vi "Fermi Level Scan.vi"() -> ()   [LabVIEW 2018]
uses:
  <vilib>/Utility/file.llb/Write Delimited Spreadsheet (string).vi
  <vilib>/Utility/file.llb/Write Delimited Spreadsheet (DBL).vi
panel:
  out "?":bool
  in  "?":bool
  in  "Log Data?":bool
  out "Supply Voltage":dbl
  out "File Location":path
  out "Electron Energy (ev)":dbl
  out "error out":errorcluster
  out "Sample Current (A)":dbl
  in  "Voltage Increment (V)":dbl(knob) scale=0.0..1.0
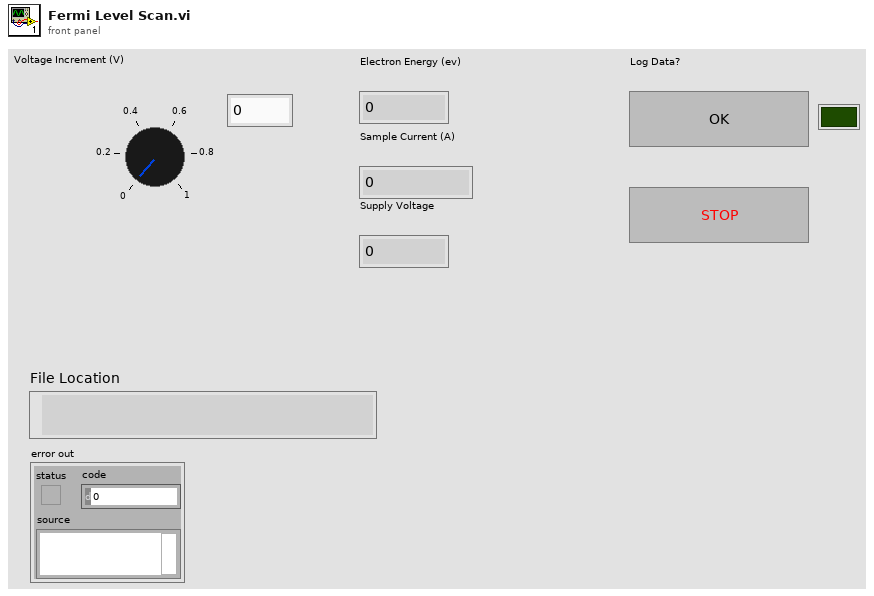
[diagram p1: front panel]
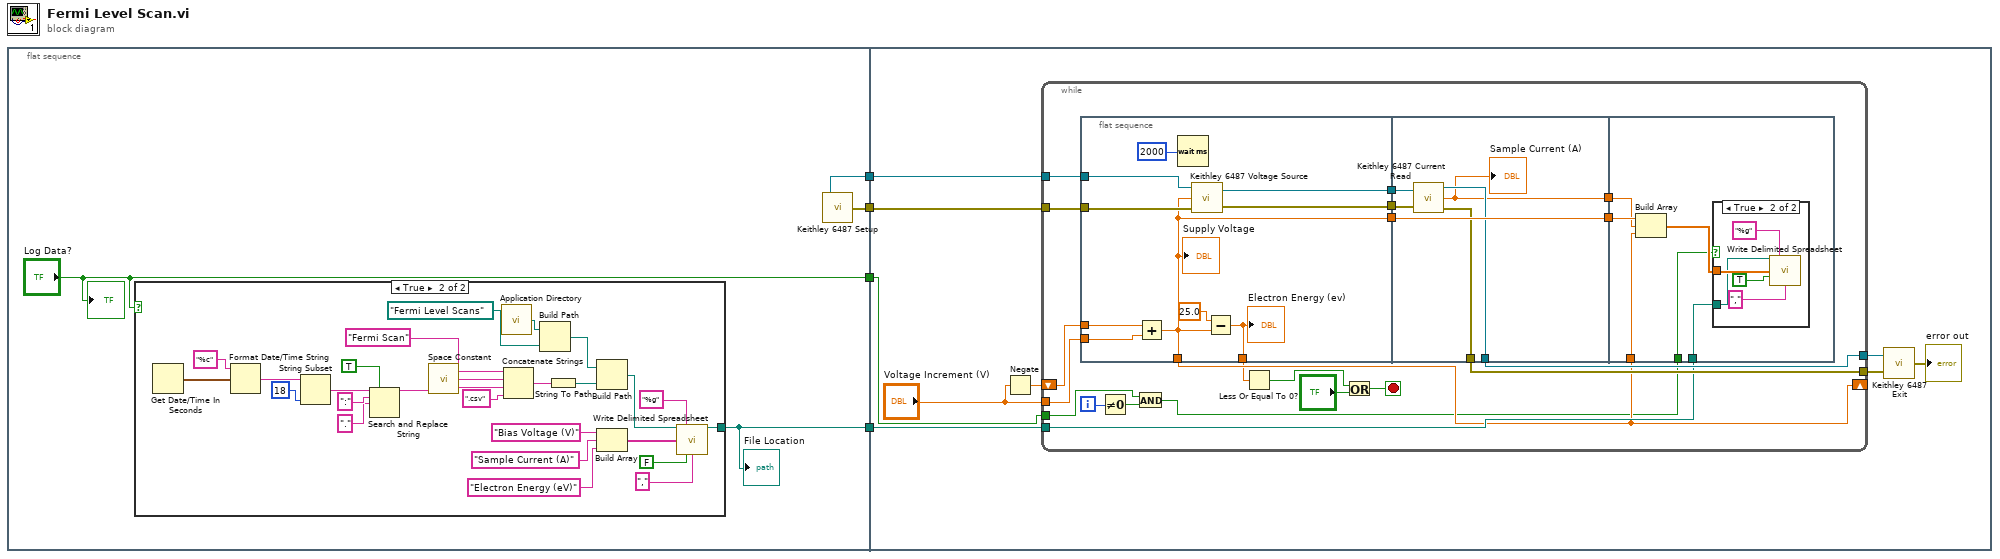
[diagram p0: block diagram]
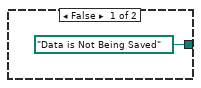
[diagram p2: hidden frame]
diagram:
  n1 = flat-sequence {
    tunnel: [w8] -> w4
    tunnel: [w6] -> w3
    tunnel: [w5] -> w2
    tunnel: ["Log Data?"] -> w1
    tunnel: w4 -> [w40]
    tunnel: w3 -> [w44]
    tunnel: w2 -> [w43]
    tunnel: w1 -> [w39]
    frame #0 {
      n2 = case shown="True" "Log Data?" {
        tunnel: [path "Data is Not Being Saved" ("new file path (Not A Path if cancelled)") w10] -> w8
        frame False {
        }
        frame True {
          n3 = Get Date/Time In Seconds() -> (seconds since 1Jan1904=w33:timestamp)
          n4 = Format Date/Time String(time format string (%c)="%c", seconds (now)=w33) -> (date/time string=w28:string)  [unwired: 1 in]
          n5 = String Subset(string=w28, length (rest)=18 ("length (rest)")) -> (substring=w29:string)  [unwired: 1 in]
          n6 = Search and Replace String(replace all?=TRUE, input string=w29, search string=":", replace string="." ("replace string (\"\")")) -> (result string=w24:string)  [unwired: 4 in, 3 out]
          n7 = call <vilib>:"Space Constant.vi"() -> ("String"=w25:string)
          n8 = call <vilib>:"Application Directory.vi"() -> ("Application Directory"=w17:path)
          n9 = Concatenate Strings("Fermi Scan", w25, w24, ".csv" ("string")) -> (w23:string)
          n10 = Build Path(base path=w17, name or relative path=path "Fermi Level Scans") -> (appended path=w34:path)
          n11 = String To Path(string=w23) -> (path=w22:path)
          n12 = Build Path(base path=w34, name or relative path=w22) -> (appended path=w21:path)
          n13 = Build Array("Bias Voltage (V)", "Sample Current (A)", "Electron Energy (eV)") -> (w12:string[])
          n14 = call-poly <vilib>:"Write Delimited Spreadsheet.vi"("file path (dialog if empty)"=w21, "format (%s)"="%g" ("format (%.3f)"), "1D data"=w12, "transpose? (no:F)"=FALSE, "delimiter (\\t)"="," ("delimiter (\\t)")) -> ("new file path (Not A Path if cancelled)"=w10:path)  [unwired: 9 in, 1 out]
        }
      }
      "File Location" <- w8
      n15 = call "Keithley 6487 Setup.vi"() -> ("error out"=w5:errorcluster, "VISA resource name out"=w6:refnum<visa-resource-name>)
      "?" <- "Log Data?"
    }
    frame #1 {
      n16 = Negate(x="Voltage Increment (V)") -> (-x=w41:dbl)
      n17 = while {
        tunnel: w44 -> [w65]
        tunnel: w43 -> [w64]
        shift-right: [w51] -> _
        shift-left: w41 -> [w61]
        tunnel: "Voltage Increment (V)" -> [w60]
        tunnel: [w58] -> w38
        tunnel: [w57] -> w37
        tunnel: w40 -> [w55]
        tunnel: w39 -> [w46]
        i -> [w48]
        stop <- w53 stop-if-true
        n18 = flat-sequence {
          tunnel: w65 -> [w68]
          tunnel: w64 -> [w69]
          tunnel: [w71] -> w63
          tunnel: [w70] -> w62
          tunnel: [w67] -> w51
          tunnel: w61 -> [w75]
          tunnel: w60 -> [w74]
          tunnel: [w67] -> w59
          tunnel: [w72] -> w50
          tunnel: w63 -> [w80]
          tunnel: w62 -> [w79]
          tunnel: w59 -> [w81]
          tunnel: [w78] -> w58
          tunnel: [w77] -> w57
          tunnel: [w81] -> w56
          tunnel: [w76] -> w52
          tunnel: w56 -> [w87]
          tunnel: w55 -> [w85]
          tunnel: w52 -> [w84]
          tunnel: w51 -> [w83]
          tunnel: w45 -> [w82]
          frame #0 {
            n19 = Add(x=w75, y=w74) -> (x+y=w67:dbl)
            "Supply Voltage" <- w67
            n20 = Wait (ms)(milliseconds to wait=u32 2000) -> ()  [unwired: 1 out]
            n21 = call "Keithley 6487 Voltage Source.vi"("error in (no error)"=w69, "Voltage"=w67, "VISA resource name"=w68) -> ("error out"=w70:errorcluster, "VISA resource name out"=w71:refnum<visa-resource-name>)
            n22 = Subtract(x=25.0, y=w67) -> (x-y=w72:dbl)
            "Electron Energy (ev)" <- w72
          }
          frame #1 {
            n23 = call "Keithley 6487 Current Read.vi"("VISA resource name"=w80, "error in (no error)"=w79) -> ("VISA out"=w78:refnum<visa-resource-name>, "Current (A)"=w76:dbl, "error out"=w77:errorcluster)
            "Sample Current (A)" <- w76
          }
          frame #2 {
            n24 = Build Array(w87, w84, w83) -> (w86:dbl[])
            n25 = case shown="True" w82 {
              tunnel: w86 -> [_ w92]
              tunnel: w85 -> [_ w91]
              frame False {
              }
              frame True {
                n26 = call-poly <vilib>:"Write Delimited Spreadsheet.vi"("file path (dialog if empty)"=w91, "format (%.3f)"="%g", "1D data"=w92, "append to file? (new file:F)"=TRUE, "delimiter (\\t)"="," ("delimiter (\\t)")) -> ()  [unwired: 9 in, 2 out]
              }
            }
          }
        }
        n27 = Not Equal To 0?(x=w48) -> (x != 0?=w47:bool)
        n28 = And(x=w46, y=w47) -> (x .and. y?=w45:bool)
        n29 = Less Or Equal To 0?(x=w50) -> (x <= 0?=w54:bool)
        n30 = Or(x=w54, y="?") -> (x .or. y?=w53:bool)
      }
      n31 = call "Keithley 6487 Exit.vi"("error in (no error)"=w37, "VISA resource name"=w38) -> ("error out"=→"error out":errorcluster)
    }
  }
